vi "Get SLSC Chassis Address.vi"(8 "error in (no error)":errorcluster, 11 "SLSC Chassis Ref in":T1 format="%.0x") -> (0 "error out":errorcluster, 1 "ChassisIDType":i32(ring) items=["ChassisName", "HostnameIPAddress"], 2 "IP Address":string, 3 "SLSC Chassis Ref out":T1 format="%.0x")   [LabVIEW 2017, in "SLSC Switch Scripting.lvlib"]
uses:
  SLSC Switch Scripting.lvlib
  <vilib>/NI Veristand/Custom Device API/Custom Device Item Ref.ctl
  NationalInstruments.VeriStand.SystemDefinitionAPI
  <vilib>/NI Veristand/Custom Device API/Custom Device API.lvlib
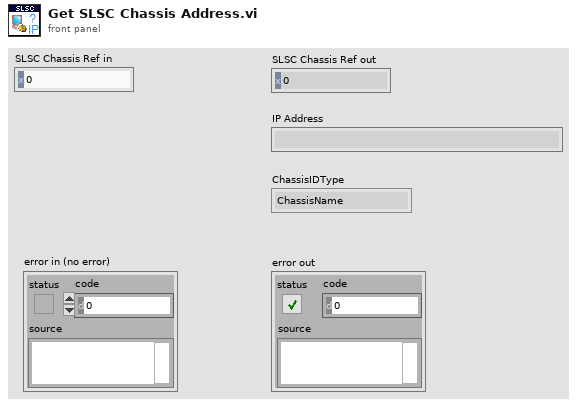
[diagram p1: front panel]
types:
  T1 = typedef "Custom Device API.lvlib/Custom Device Item Ref.ctl" = u64
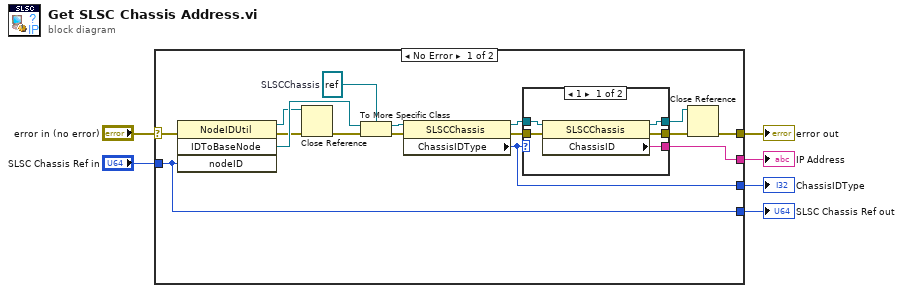
[diagram p0: block diagram]
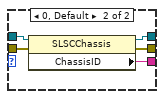
[diagram p2: hidden frame]
diagram:
  n1 = case shown="No Error" "error in (no error)" {
    selector: "error in (no error)" -> [w8 w34]
    tunnel: [w22 _] -> w6
    tunnel: [w16 w34] -> w5
    tunnel: [w9 _] -> w4
    tunnel: "SLSC Chassis Ref in" -> [w7 w33]
    tunnel: [w7 w33] -> w1
    frame No Error {
      w21 = refnum<k24> refnum  # SLSCChassis
      n2 = invoke class="NodeIDUtil" method="IDToBaseNode"(error in=w8, "nodeID"=w7) -> (reference out=w17:refnum<k24>, error out=w18:errorcluster, "IDToBaseNode"=w20:refnum<k24>)  [unwired: 2 in, 1 out]
      n3 = Close Reference(reference=w17, error in (no error)=w18) -> (error out=w19:errorcluster)
      n4 = To More Specific Class(target class=w21, reference=w20, error in=w19) -> (specific class reference=w15:refnum<k24>, error out=w14:errorcluster)
      n5 = property class="SLSCChassis"(reference=w15, error in=w14) -> (reference out=w13:refnum<k24>, error out=w12:errorcluster, "ChassisIDType"=w9:i32)
      n6 = case shown="1" w9 {
        tunnel: [w27 w32] -> w22
        tunnel: w13 -> [w26 w31]
        tunnel: w12 -> [w25 w30]
        tunnel: [w24 w29] -> w11
        tunnel: [w23 w28] -> w10
        frame 1 {
          n7 = property class="SLSCChassis"(reference=w26, error in=w25) -> (reference out=w24:refnum<k24>, error out=w23:errorcluster, "ChassisID"=w27:string)
        }
        frame 0, Default {
          n8 = property class="SLSCChassis"(reference=w31, error in=w30) -> (reference out=w29:refnum<k24>, error out=w28:errorcluster, "ChassisID"=w32:string)
        }
      }
      n9 = Close Reference(reference=w11, error in (no error)=w10) -> (error out=w16:errorcluster)
    }
    frame Error {
    }
  }
  "ChassisIDType" <- w4
  "error out" <- w5
  "IP Address" <- w6
  "SLSC Chassis Ref out" <- w1
